vi "camera get one frame-subvi.vi"(2 "error in":errorcluster, 3 "New Image":T2, 4 "Image Size":T1 {"V Bin" min=0.0; "H Bin" min=0.0 step=1.0}) -> (0 "error out":errorcluster, 1 "Image Out":T2)   [LabVIEW 2014]
uses:
  <vilib>/vision/Image Controls.llb/IMAQ Image.ctl
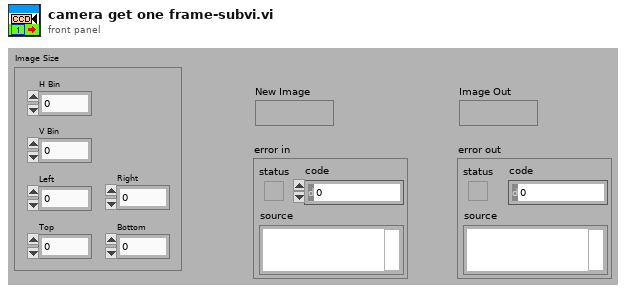
[diagram p1: front panel]
types:
  T1 = cluster{"H Bin":dbl, "V Bin":dbl, "Left":dbl, "Right":dbl, "Top":dbl, "Bottom":dbl}
  T2 = typedef "IMAQ Image.ctl" = refnum<image>
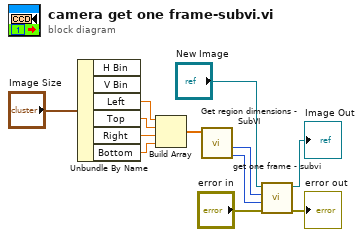
[diagram p0: block diagram]
diagram:
  n1 = Unbundle By Name("Image Size") -> ("Left"=w11:dbl, "Top"=w10:dbl, "Right"=w9:dbl, "Bottom"=w8:dbl)  [unwired: 2 out]
  n2 = Build Array(w11, w10, w9, w8) -> (w12:dbl[])
  n3 = call "Get region dimensions - SubVI.vi"("x1y1x2y2"=w12) -> ("y size"=w3:u16, "x size"=w4:u16)  [unwired: 7 in, 2 out]
  n4 = call "get one frame - subvi.vi"("error in"="error in", "Image Height"=w3, "Image Width"=w4, "Image In"="New Image") -> ("error out"=→"error out":errorcluster, "Image Out"=→"Image Out":T2)  [unwired: 6 in]
